vi "module-07-sample-7-1.vi"() -> ()   [LabVIEW 2019]
uses:
  <vilib>/Rock Robotics/WPI/ThirdParty/JAS_Junk/TrajLib/Trajectory_Library.lvlib
  samples-common-library/Ctrl_Training_Library_Protected/CtrlTrainingLibary_Protected.lvlib
panel:
  in  "Tab Control":T1(tab)
  in  "Driver Gather Cube":bool
  in  "Driver Cancel Button":bool
  out "Request GO":bool
  out "Digital State Chart":cluster{dbl, dbl, dbl, dbl, dbl, dbl}(graph)
  out "Ready":bool
  out "Arm Extend Cmd":bool
  out "Hand Close Cmd":bool
  out "State":dbl
  out "Done Time":dbl format="%20.3f"
  out "Cur Time":dbl format="%20.3f"
  # "Training Sample 7.1\nState Machine"
  # "F1"
  # "F2"
  # "Other Conditonal States"
  # "Other Conditonal States"
  # "Other Conditonal States"
  # "Other Conditonal States"
  # "Other Conditonal States"
  # "Other Conditonal States"
  # "Other Conditonal States"
  # "Other Conditonal States"
  # "Other Conditonal States"
  # "Other Conditonal States"
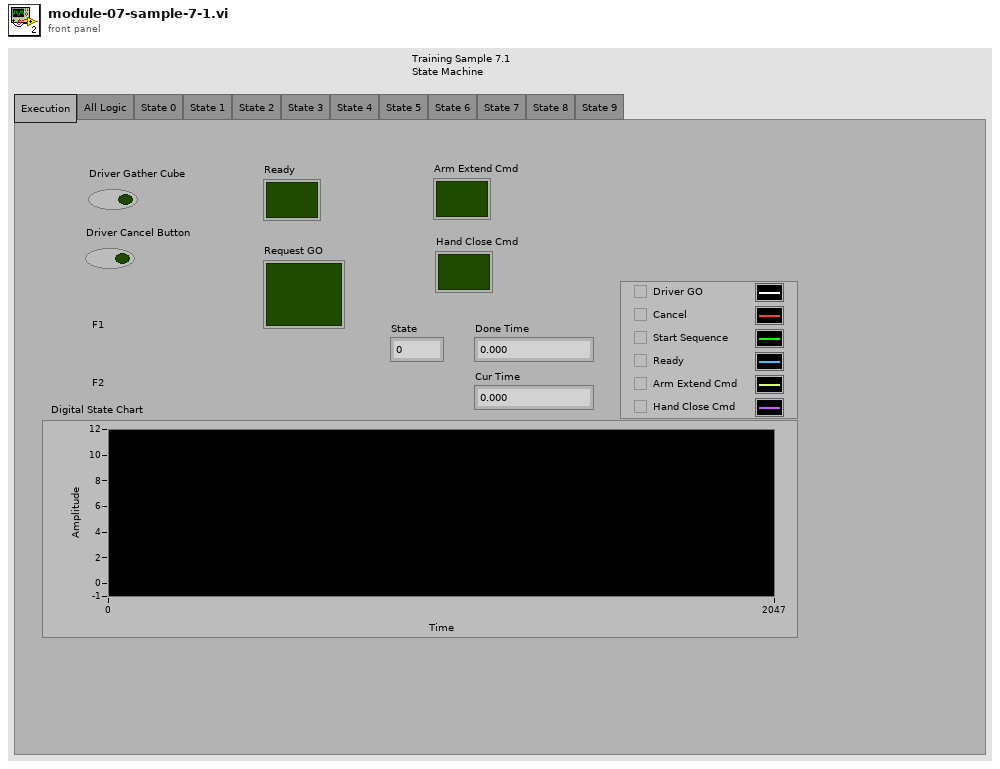
[diagram p1: front panel]
types:
  T1 = enum32{"Execution", "All Logic", "State 0", "State 1", "State 2", "State 3", "State 4", "State 5", "State 6", "State 7", "State 8", "State 9"}
  T2 = typedef "Trajectory_Library.lvlib/TIMER.ctl" = cluster{"StartTime":dbl, "Accumulated TIme":dbl, "Running":bool, "semaphore":T3}
  T3 = typedef "Semaphore RefNum" = refnum<k1>
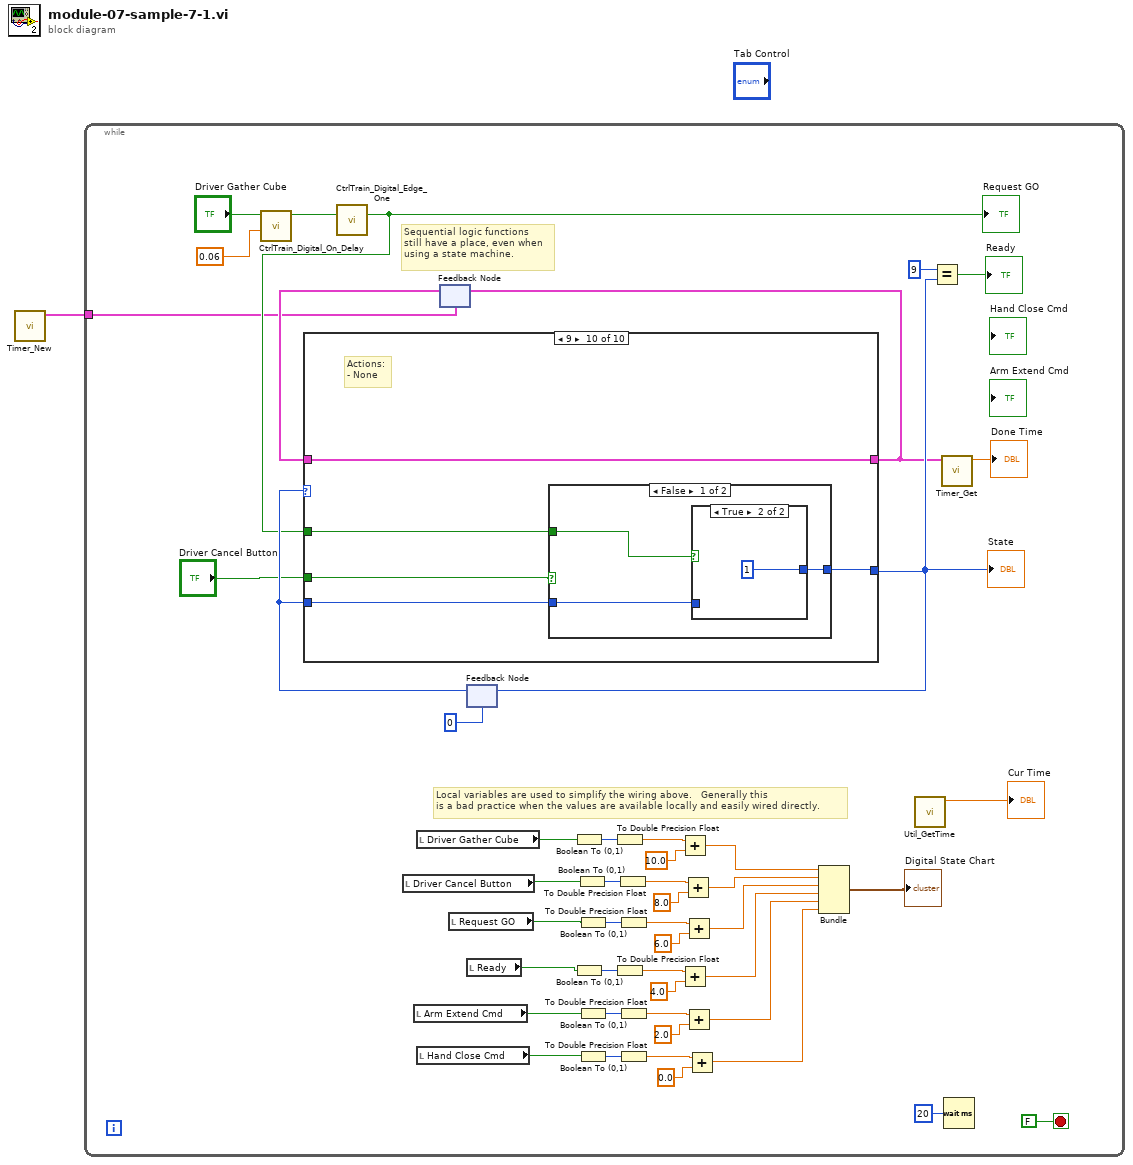
[diagram p0: block diagram]
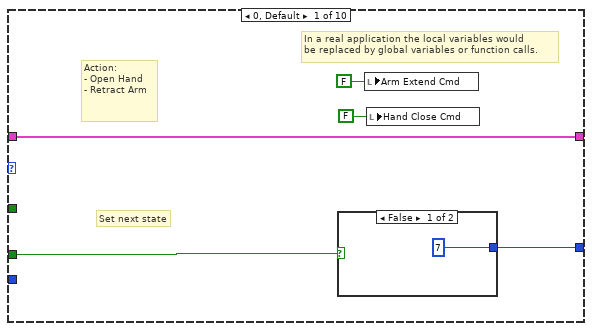
[diagram p2: hidden frame]
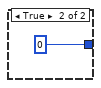
[diagram p3: hidden frame]
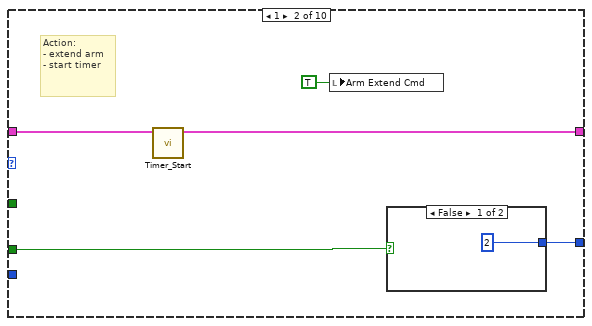
[diagram p4: hidden frame]
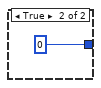
[diagram p5: hidden frame]
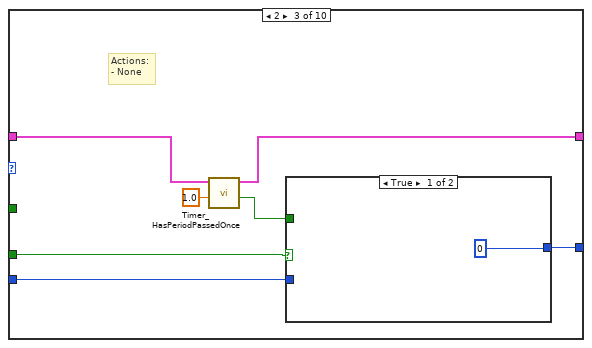
[diagram p6: hidden frame]
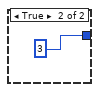
[diagram p8: hidden frame]
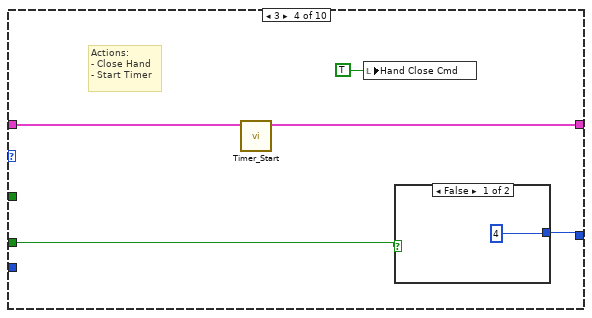
[diagram p9: hidden frame]
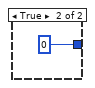
[diagram p10: hidden frame]
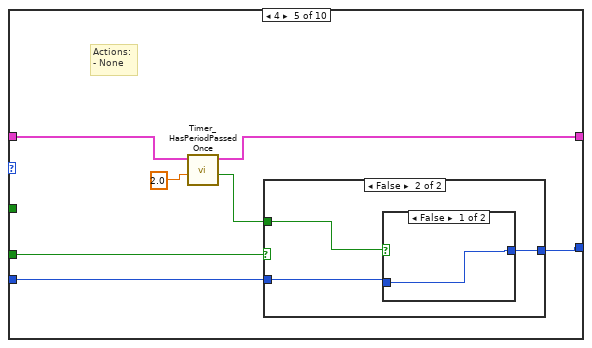
[diagram p11: hidden frame]
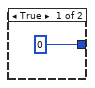
[diagram p12: hidden frame]
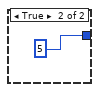
[diagram p13: hidden frame]
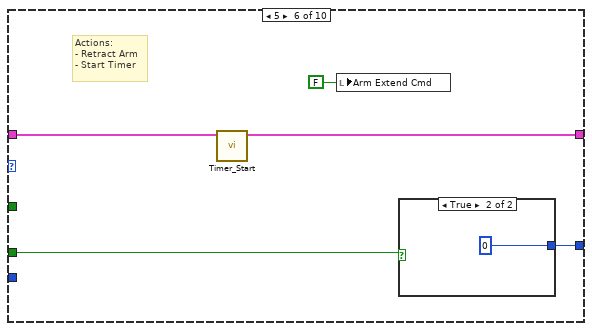
[diagram p14: hidden frame]
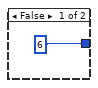
[diagram p15: hidden frame]
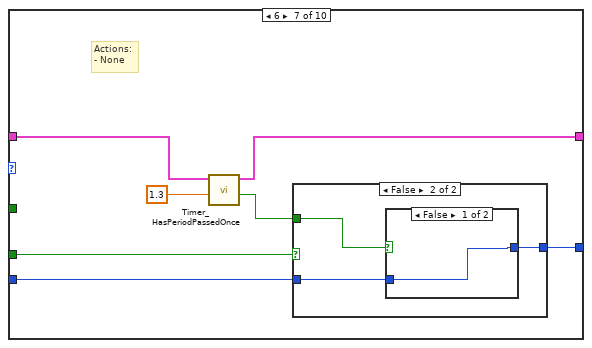
[diagram p16: hidden frame]
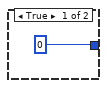
[diagram p17: hidden frame]
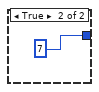
[diagram p18: hidden frame]
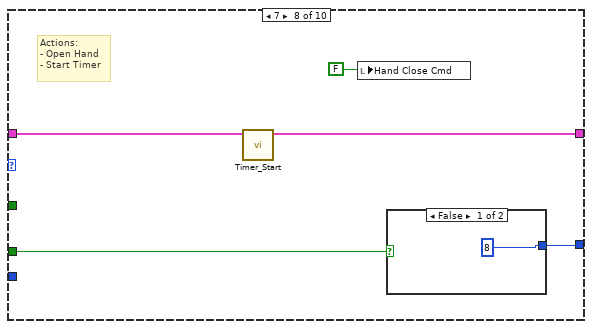
[diagram p19: hidden frame]
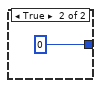
[diagram p20: hidden frame]
diagram:
  n1 = call <vilib>:"Timer_New.vi"() -> ("TIMER"=w1:T2)  [unwired: 11 in]
  n2 = while {
    tunnel: w1 -> [w7]
    stop <- FALSE stop-if-true
    # "Sequential logic functions\nstill have a place, even when\nusing a state machine."
    # "Local variables are used to simplify the wiring above.   Generally this\nis a bad practice when the values are available locally and easily wired directly."
    n3 = call "CtrlTrain_Digital_On_Delay.vi"("Delay"=0.06, "Input"="Driver Gather Cube") -> ("Output"=w14:bool)  [unwired: 8 in, 1 out]
    n4 = call "CtrlTrain_Digital_Edge_One.vi"("Input"=w14) -> ("Output"=w8:bool)  [unwired: 14 in]
    "Request GO" <- w8
    n5 = local read "Driver Cancel Button"() -> (w3:bool)
    n6 = local read "Arm Extend Cmd"() -> (w21:bool)
    n7 = local read "Driver Gather Cube"() -> (w2:bool)
    n8 = local read "Hand Close Cmd"() -> (w22:bool)
    n9 = feedback #1(w7) -> (w17:T2)
    n10 = local read "Request GO"() -> (w20:bool)
    n11 = feedback #2(u32 0) -> (w11:u32)
    n12 = case shown="9" w11 {
      tunnel: [w51 w58 w69 w81 w90 w101 w110 w121 w130 w140] -> w10
      tunnel: [w52 w59 w65 w77 w85 w98 w106 w117 w125 w141] -> w5
      tunnel: w17 -> [w52 w60 w67 w78 w86 w97 w107 w118 w127 w141]
      tunnel: w11 -> [_ _ w70 _ w89 _ w109 _ w129 w139]
      tunnel: "Driver Cancel Button" -> [w50 w57 w68 w79 w88 w99 w108 w119 w128 w138]
      tunnel: w8 -> [_ _ _ _ _ _ _ _ _ w137]
      frame 0, Default {
        # "In a real application the local variables would\nbe replaced by global variables or function calls."
        # "Set next state"
        # "Action:\n- Open Hand \n- Retract Arm"
        n13 = case shown="False" w50 {
          tunnel: [u32 7 u32 0] -> w51
          frame False {
          }
          frame True {
          }
        }
        n14 = local write "Arm Extend Cmd"(FALSE ("Arm Extend Cmd")) -> ()
        n15 = local write "Hand Close Cmd"(FALSE ("Hand Close Cmd")) -> ()
      }
      frame 1 {
        # "Action:\n- extend arm \n- start timer"
        n16 = call <vilib>:"Timer_Start.vi"("in Timer"=w60) -> ("out Timer"=w59:T2)  [unwired: 10 in]
        n17 = local write "Arm Extend Cmd"(TRUE ("Arm Extend Cmd")) -> ()
        n18 = case shown="False" w57 {
          tunnel: [u32 2 u32 0] -> w58
          frame False {
          }
          frame True {
          }
        }
      }
      frame 2 {
        # "Actions:\n- None"
        n19 = call <vilib>:"Timer_HasPeriodPassedOnce.vi"("Period"=1.0, "in Timer"=w67) -> ("Expired"=w64:bool, "out Timer"=w65:T2)  [unwired: 7 in, 1 out]
        n20 = case shown="True" w68 {
          tunnel: w70 -> [_ w74]
          tunnel: w64 -> [_ w73]
          tunnel: [u32 0 w72] -> w69
          frame True {
          }
          frame False {
            n21 = case shown="False" w73 {
              tunnel: w74 -> [w75 _]
              tunnel: [w75 u32 3] -> w72
              frame False {
              }
              frame True {
              }
            }
          }
        }
      }
      frame 3 {
        # "Actions:\n- Close Hand\n- Start Timer"
        n22 = call <vilib>:"Timer_Start.vi"("in Timer"=w78) -> ("out Timer"=w77:T2)  [unwired: 10 in]
        n23 = local write "Hand Close Cmd"(TRUE ("Hand Close Cmd")) -> ()
        n24 = case shown="False" w79 {
          tunnel: [u32 4 u32 0] -> w81
          frame False {
          }
          frame True {
          }
        }
      }
      frame 4 {
        # "Actions:\n- None"
        n25 = call <vilib>:"Timer_HasPeriodPassedOnce.vi"("Period"=2.0 ("Elapsed"), "in Timer"=w86) -> ("Expired"=w84:bool, "out Timer"=w85:T2)  [unwired: 7 in, 1 out]
        n26 = case shown="False" w88 {
          tunnel: w84 -> [_ w94]
          tunnel: [u32 0 w93] -> w90
          tunnel: w89 -> [_ w92]
          frame True {
          }
          frame False {
            n27 = case shown="False" w94 {
              tunnel: w92 -> [w95 _]
              tunnel: [w95 u32 5] -> w93
              frame False {
              }
              frame True {
              }
            }
          }
        }
      }
      frame 5 {
        # "Actions:\n- Retract Arm\n- Start Timer"
        n28 = call <vilib>:"Timer_Start.vi"("in Timer"=w97) -> ("out Timer"=w98:T2)  [unwired: 10 in]
        n29 = local write "Arm Extend Cmd"(FALSE ("Arm Extend Cmd")) -> ()
        n30 = case shown="True" w99 {
          tunnel: [u32 6 u32 0] -> w101
          frame False {
          }
          frame True {
          }
        }
      }
      frame 6 {
        # "Actions:\n- None"
        n31 = call <vilib>:"Timer_HasPeriodPassedOnce.vi"("Period"=1.3 ("Elapsed"), "in Timer"=w107) -> ("Expired"=w104:bool, "out Timer"=w106:T2)  [unwired: 7 in, 1 out]
        n32 = case shown="False" w108 {
          tunnel: w104 -> [_ w114]
          tunnel: [u32 0 w113] -> w110
          tunnel: w109 -> [_ w112]
          frame True {
          }
          frame False {
            n33 = case shown="False" w114 {
              tunnel: w112 -> [w115 _]
              tunnel: [w115 u32 7] -> w113
              frame False {
              }
              frame True {
              }
            }
          }
        }
      }
      frame 7 {
        # "Actions:\n- Open Hand\n- Start Timer"
        n34 = call <vilib>:"Timer_Start.vi"("in Timer"=w118) -> ("out Timer"=w117:T2)  [unwired: 10 in]
        n35 = local write "Hand Close Cmd"(FALSE ("Hand Close Cmd")) -> ()
        n36 = case shown="False" w119 {
          tunnel: [u32 8 u32 0] -> w121
          frame False {
          }
          frame True {
          }
        }
      }
      frame 8 {
        # "Actions:\n- None"
        n37 = call <vilib>:"Timer_HasPeriodPassedOnce.vi"("Period"=1.5 ("Elapsed"), "in Timer"=w127) -> ("Expired"=w126:bool, "out Timer"=w125:T2)  [unwired: 7 in, 1 out]
        n38 = case shown="False" w128 {
          tunnel: w126 -> [_ w134]
          tunnel: [u32 0 w133] -> w130
          tunnel: w129 -> [_ w132]
          frame True {
          }
          frame False {
            n39 = case shown="True" w134 {
              tunnel: w132 -> [w135 _]
              tunnel: [w135 u32 9] -> w133
              frame False {
              }
              frame True {
              }
            }
          }
        }
      }
      frame 9 {
        # "Actions:\n- None"
        n40 = case shown="False" w138 {
          tunnel: [w144 u32 0] -> w140
          tunnel: w139 -> [w143 _]
          tunnel: w137 -> [w142 _]
          frame False {
            n41 = case shown="True" w142 {
              tunnel: [w145 u32 1] -> w144
              tunnel: w143 -> [w145 _]
              frame False {
              }
              frame True {
              }
            }
          }
          frame True {
          }
        }
      }
    }
    "State" <- w10
    n42 = feedback-in #1(w5) -> ()
    n43 = feedback-in #2(w10) -> ()
    n44 = local read "Ready"() -> (w19:bool)
    n45 = Boolean To (0,1)(Boolean=w2) -> (0, 1=w47:i16)
    n46 = Boolean To (0,1)(Boolean=w19) -> (0, 1=w45:i16)
    n47 = Boolean To (0,1)(Boolean=w3) -> (0, 1=w42:i16)
    n48 = Boolean To (0,1)(Boolean=w20) -> (0, 1=w39:i16)
    n49 = Boolean To (0,1)(Boolean=w21) -> (0, 1=w36:i16)
    n50 = Boolean To (0,1)(Boolean=w22) -> (0, 1=w33:i16)
    n51 = To Double Precision Float(number=w47) -> (double precision float=w24:dbl)
    n52 = To Double Precision Float(number=w45) -> (double precision float=w44:dbl)
    n53 = To Double Precision Float(number=w42) -> (double precision float=w41:dbl)
    n54 = To Double Precision Float(number=w39) -> (double precision float=w38:dbl)
    n55 = To Double Precision Float(number=w36) -> (double precision float=w35:dbl)
    n56 = To Double Precision Float(number=w33) -> (double precision float=w32:dbl)
    n57 = Add(x=w24, y=10.0) -> (x+y=w23:dbl)
    n58 = Add(x=w44, y=4.0) -> (x+y=w27:dbl)
    n59 = Add(x=w41, y=8.0) -> (x+y=w29:dbl)
    n60 = Add(x=w38, y=6.0) -> (x+y=w28:dbl)
    n61 = Add(x=w35, y=2.0) -> (x+y=w31:dbl)
    n62 = Add(x=w32, y=0.0) -> (x+y=w30:dbl)
    n63 = Bundle(w23, w29, w28, w27, w31, w30) -> (→"Digital State Chart":cluster{dbl, dbl, dbl, dbl, dbl, dbl})  [unwired: 1 in]
    n64 = call <vilib>:"Util_GetTime.vi"() -> ("FPGA_Time_Seconds"=→"Cur Time":dbl)  [unwired: 10 in, 1 out]
    n65 = Equal?(x=u32 9, y=w10) -> (x = y?=→"Ready":bool)
    n66 = call <vilib>:"Timer_Get.vi"("TIMER"=w5) -> ("CurrentTImer"=→"Done Time":dbl)  [unwired: 10 in]
    n67 = Wait (ms)(milliseconds to wait=u32 20) -> ()  [unwired: 1 out]
  }
